vi "WPI_MotorControlSafetyError.vi"(0 "MotorControlDevRef":T1={"DeviceStatus"={"status"=FALSE, "code"=0, "source"=""}, "Type"=enum."PWM", "PWM"={"PWM Channel"=enum."Invalid", "DeadBand"={"Name"="", "maxPositivePwm"=0, "minPositivePwm"=0, "centerPwm"=0, "maxNegativePwm"=0, "minNegativePwm"=0, "angularRange"=0}}, "CAN"={"Device Number"=0, "SetOutput VI Ref"=variant(refnum<vi> refnum), "GetOutput VI Ref"=variant(refnum<vi> refnum), "Enable VI Ref"=variant(refnum<vi> refnum), "Disable VI Ref"=variant(refnum<vi> refnum), "Data"=variant}, "Invert"=FALSE, "DIO PWM"={"PWM \"Enable\" Channel"=enum."Invalid", "DIOChannel"=enum."Invalid", "PWM Rate"=0.0}}) -> (4 "MotorControlDevRef":T1={"DeviceStatus"={"status"=FALSE, "code"=0, "source"=""}, "Type"=enum."PWM", "PWM"={"PWM Channel"=enum."Invalid", "DeadBand"={"Name"="", "maxPositivePwm"=0, "minPositivePwm"=0, "centerPwm"=0, "maxNegativePwm"=0, "minNegativePwm"=0, "angularRange"=0}}, "CAN"={"Device Number"=0, "SetOutput VI Ref"=variant(refnum<vi> refnum), "GetOutput VI Ref"=variant(refnum<vi> refnum), "Enable VI Ref"=variant(refnum<vi> refnum), "Disable VI Ref"=variant(refnum<vi> refnum), "Data"=variant}, "Invert"=FALSE, "DIO PWM"={"PWM \"Enable\" Channel"=enum."Invalid", "DIOChannel"=enum."Invalid", "PWM Rate"=0.0}})   [LabVIEW 2025]
doc: "This subVI does two things:\n1. It builds up output specific information to help locate the problem.\n2. It calls the FRC Build Error, so all the information gets passed to the Driver Station."
uses:
  <vilib>/Rock Robotics/WPI/MotorControl/WPI_MotorControlDeviceRef.ctl
  <vilib>/Rock Robotics/WPI/MotorControl/WPI_MotorControlType.ctl
  <vilib>/Rock Robotics/SystemInterfaces/DIO/FPGA_DIOPWMChannel.ctl
  <vilib>/Rock Robotics/WPI/PWM/WPI_PWMDeadband.ctl
  <vilib>/Rock Robotics/SystemInterfaces/DIO/FPGA_DIOChannel.ctl
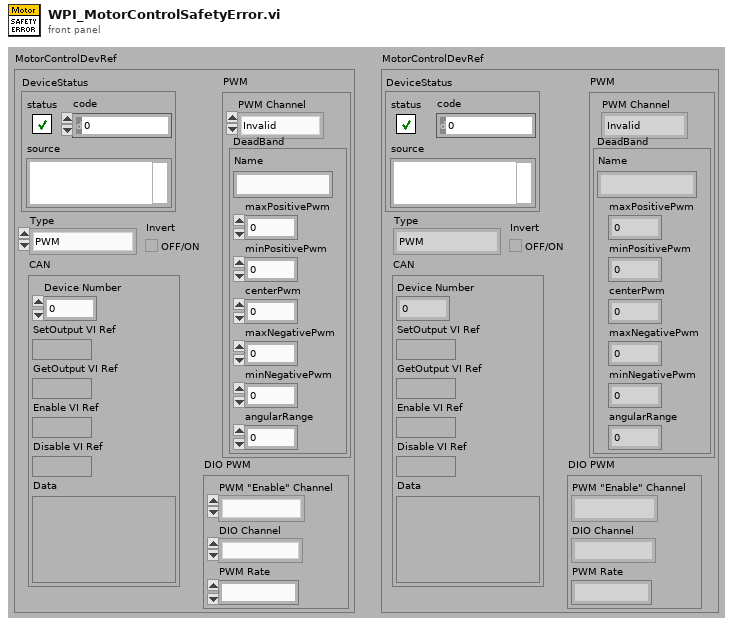
[diagram p1: front panel]
types:
  T1 = typedef "WPI_MotorControlDeviceRef.ctl" = cluster{"DeviceStatus":errorcluster, "Type":T2, "PWM":cluster{"PWM Channel":T3, "DeadBand":T4}, "CAN":cluster{"Device Number":u8, "SetOutput VI Ref":variant, "GetOutput VI Ref":variant, "Enable VI Ref":variant, "Disable VI Ref":variant, "Data":variant}, "Invert":bool, "DIO PWM":cluster{"PWM \"Enable\" Channel":T3, "DIOChannel":T5, "PWM Rate":dbl}}
  T2 = typedef "WPI_MotorControlType.ctl" = enum16{"PWM", "CAN", "DIO PWM"}
  T3 = typedef "FPGA_DIOPWMChannel.ctl" = enum8{"PWM 0", "PWM 1", "PWM 2", "PWM 3", "PWM 4", "PWM 5", "PWM 6", "PWM 7", "PWM 8", "PWM 9", "PWM MXP 0", "PWM MXP 1", "PWM MXP 2", "PWM MXP 3", "PWM MXP 4", "PWM MXP 5", "PWM MXP 6", "PWM MXP 7", "PWM MXP 8", "PWM MXP 9", "Invalid"}
  T4 = typedef "WPI_PWMDeadband.ctl" = cluster{"Name":string, "maxPositivePwm":i32, "minPositivePwm":i32, "centerPwm":i32, "maxNegativePwm":i32, "minNegativePwm":i32, "angularRange":u16}
  T5 = typedef "FPGA_DIOChannel.ctl" = enum8{"DIO 0", "DIO 1", "DIO 2", "DIO 3", "DIO 4", "DIO 5", "DIO 6", "DIO 7", "DIO 8", "DIO 9", "DIO MXP 0", "DIO MXP 1", "DIO MXP 2", "DIO MXP 3", "DIO MXP 4", "DIO MXP 5", "DIO MXP 6", "DIO MXP 7", "DIO MXP 8", "DIO MXP 9", "DIO MXP 10", "DIO MXP 11", "DIO MXP 12", "DIO MXP 13", "DIO MXP 14", "DIO MXP 15", "SPI Port CS1", "SPI Port CS2", "SPI Port CS3", "SPI Port MISO", "SPI Port MOSI", "Invalid"}
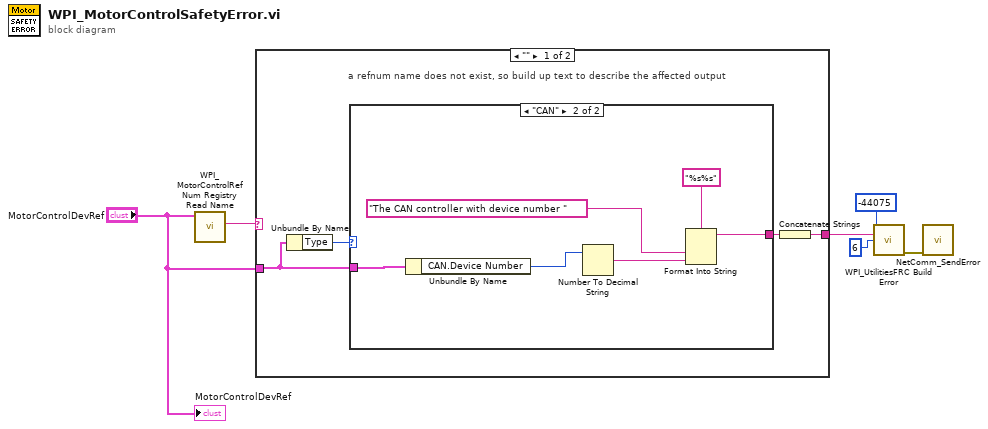
[diagram p0: block diagram]
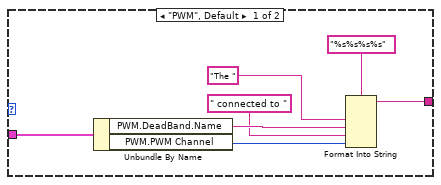
[diagram p2: hidden frame]
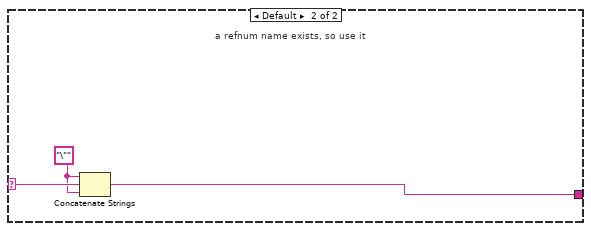
[diagram p3: hidden frame]
diagram:
  n1 = call <vilib>:"WPI_MotorControlRefNum Registry Read Name.vi"("MotorControlDeviceRef"="MotorControlDevRef") -> ("refnum name"=w4:string)  [unwired: 1 in, 9 out]
  n2 = case shown="\"\"" w4 {
    selector: w4 -> [_ w26]
    tunnel: [w9 w25] -> w3
    tunnel: "MotorControlDevRef" -> [w8 _]
    frame "" {
      # "a refnum name does not exist, so build up text to describe the affected output"
      n3 = Unbundle By Name(w8) -> ("Type"=w7:T2)
      n4 = case shown="\"CAN\"" w7 {
        tunnel: [w17 w21] -> w10
        tunnel: w8 -> [w11 w20]
        frame "PWM", Default {
          n5 = Unbundle By Name(w11) -> ("PWM.DeadBand.Name"=w15:string, "PWM.PWM Channel"=w13:T3)
          n6 = Format Into String(format string="%s%s%s%s", "The " ("format string"), w15, " connected to " ("format string"), w13) -> (resulting string=w17:string)  [unwired: 2 in, 1 out]
        }
        frame "CAN" {
          n7 = Unbundle By Name(w20) -> ("CAN.Device Number"=w18:u8)
          n8 = Number To Decimal String(number=w18) -> (decimal integer string=w19:string)  [unwired: 1 out]
          n9 = Format Into String(format string="%s%s", "The CAN controller with device number " ("format string"), w19) -> (resulting string=w21:string)  [unwired: 2 in, 1 out]
        }
      }
      n10 = Concatenate Strings(w10) -> (w9:string)
    }
    frame Default {
      w24 = "\"" ("string")
      # "a refnum name exists, so use it"
      n11 = Concatenate Strings(w24, w26, w24) -> (w25:string)
    }
  }
  n12 = call <vilib>:"WPI_UtilitiesFRC Build Error.vi"("error code"=-44075 ("code"), "extra error text"=w3, "chain levels to remove (1)"=6) -> ("error out"=w1:errorcluster)  [unwired: 3 in, 9 out]
  n13 = call <vilib>:"NetComm_SendError.vi"("error in (no error)"=w1) -> ()  [unwired: 11 in]
  "MotorControlDevRef" <- "MotorControlDevRef"
